vi "Test Function 1.vi"(1 "x":refnum<class "Dual.lvclass">) -> (0 "f(x)":refnum<class "Dual.lvclass">)   [LabVIEW 2020, in "Tests.lvlib"]
uses:
  Tests.lvlib
  classes/Dual/Dual.lvclass
  classes/Dual/Dual.lvclass/Dual.ctl
  9ee1d76c-c68c-43aa-a686-36ea2697e5af.vi
  2339b2d4-4176-426a-a400-f0798d2c3531.vi
  06373cf3-2925-40e9-b0a2-8989fd62f293.vi
  7805c8b1-a590-4d51-98fb-eb1755892a98.vi
  1dc40f4b-cd1a-4eea-ab3f-554bb7f0e0e1.vi
  9ee1d76c-c68c-43aa-a686-36ea2697e5af.vi/5957e011-cf56-4527-b6ed-13c3a4ca997b.vi
  classes/Dual/Write a.vi
  2339b2d4-4176-426a-a400-f0798d2c3531.vi/968883c3-f1f3-473a-bfc5-8cde3e5b01f7.vi
  2339b2d4-4176-426a-a400-f0798d2c3531.vi/bec82738-76c0-439a-a1c7-54fdd631a6e8.vi
  classes/Dual/Read a and b.vi
  classes/Dual/Write a and b.vi
  06373cf3-2925-40e9-b0a2-8989fd62f293.vi/957074e8-cc3b-4647-8ff1-d975a744cd4e.vi
  7805c8b1-a590-4d51-98fb-eb1755892a98.vi/957074e8-cc3b-4647-8ff1-d975a744cd4e.vi
  1dc40f4b-cd1a-4eea-ab3f-554bb7f0e0e1.vi/b6499733-2759-4852-aa6b-3ec1516ef704.vi
  1dc40f4b-cd1a-4eea-ab3f-554bb7f0e0e1.vi/ce7907ec-4dc6-4618-8708-ad667a8e3a23.vi
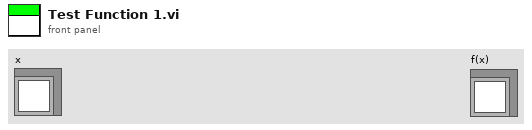
[diagram p1: front panel]
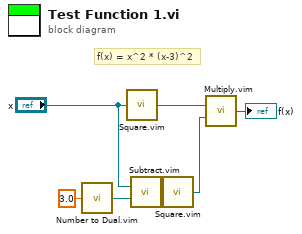
[diagram p0: block diagram]
diagram:
  # "f(x) = x^2 * (x-3)^2"
  n1 = call "Number to Dual.vim"("Number"=3.0 ("a")) -> ("Dual"=w4:refnum<class "Dual.lvclass">)
  n2 = call "Square.vim"("x"="x") -> ("x^2"=w3:refnum<class "Dual.lvclass">)
  n3 = call "Subtract.vim"("x"="x", "y"=w4) -> ("x - y"=w6:refnum<class "Dual.lvclass">)  [unwired: 13 in]
  n4 = call "Square.vim"("x"=w6) -> ("x^2"=w2:refnum<class "Dual.lvclass">)
  n5 = call "Multiply.vim"("x"=w3, "y"=w2) -> ("x * y"=→"f(x)":refnum<class "Dual.lvclass">)  [unwired: 13 in]
